vi "Arduino DAQ LabVIEW.vi"() -> ()   [LabVIEW 2020]
uses:
  <vilib>/MakerHub/LINX/Public/Peripherals/Analog/Analog Read N Chans.vi
  <vilib>/MakerHub/LINX/Public/Peripherals/Analog/Analog Read 1 Chan.vi
  <vilib>/MakerHub/LINX/Private/Local IO/LinxAnalogRead.vi
  <vilib>/MakerHub/LINX/Public/Utilities/Check Channel.vi
  <vilib>/MakerHub/LINX/Public/Utilities/Open Serial.vi
  <vilib>/MakerHub/LINX/Private/Utilties/Generate Error.vi
  <vilib>/MakerHub/LINX/LMH-LINX.lvlib
panel:
  out "Voltages":dbl[](array[numeric])
  in  "AI Channel(s)":u8[](array[numeric])
  out "Waveform Chart":dbl(graph)
  out "Voltage":dbl
  in  "Serial Port":refnum<visa-resource-name>="N/A"
  in  "Stop":bool
  in  "Analog Channel":u8
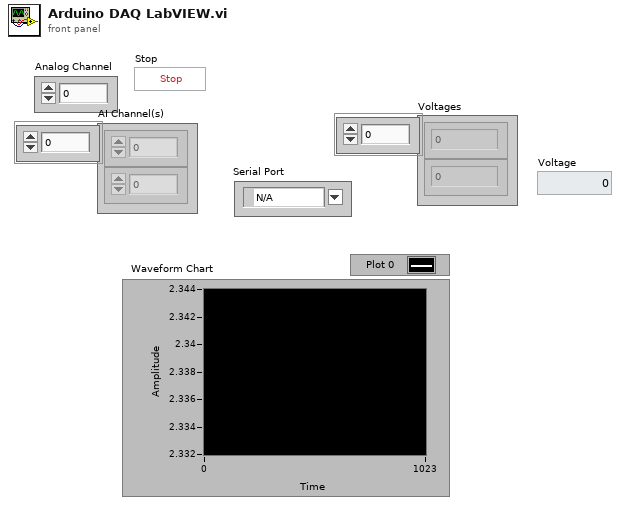
[diagram p1: front panel]
types:
  T1 = typedef "LMH-LINX.lvlib/LINX Ref.ctl" = cluster{"IO":T2, "Interface":T3, "LINX Device Config":T4}
  T2 = typedef "LMH-LINX.lvlib/Platform.ctl" = enum16{"Remote", "Local"}
  T3 = typedef "LMH-LINX.lvlib/Interface.ctl" = enum16{"Serial", "TCP"}
  T4 = typedef "LMH-LINX.lvlib/Device.lvlib/LINX Device Config.ctl" = cluster{"Interface":T3, "COM Port":refnum<visa-resource-name>, "TCP Configuration":T5, "Device Family":u8, "Device ID":u8, "Device Name":string, "TCP Ref":refnum<k5>, "Channels":T6}
  T5 = typedef "LMH-LINX.lvlib/Device.lvlib/TCP Config.ctl" = cluster{"IP Address":string, "Port":u16}
  T6 = typedef "LMH-LINX.lvlib/Channels.ctl" = cluster{"DI":u8[], "DO":u8[], "AI":u8[], "AO":u8[], "PWM":u8[], "QE":u8[], "UART":u8[], "I2C 2":u8[], "SPI":u8[], "CAN":u8[], "Servo":u8[], "AI Ref (V)":dbl, "AI Resolution (Bits)":u8, "AO Ref (V)":dbl, "AO Resolution (Bits)":u8}
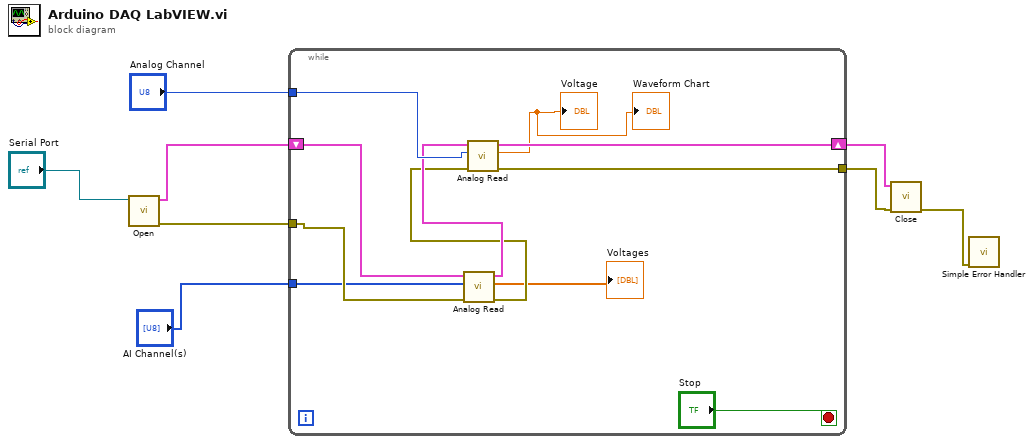
[diagram p0: block diagram]
diagram:
  n1 = call-poly <vilib>:"Open.vi"("Serial Port"="Serial Port") -> ("Error Out"=w7:errorcluster, "LINX Resource"=w8:T1)  [unwired: 8 in, 1 out]
  n2 = while {
    tunnel: w7 -> [w16]
    tunnel: "Analog Channel" -> [w18]
    tunnel: [w14] -> w2
    tunnel: "AI Channel(s)" -> [w10]
    shift-right: [w15] -> w3
    shift-left: w8 -> [w17]
    stop <- "Stop" stop-if-true
    n3 = call-poly <vilib>:"Analog Read.vi"("Error In"=w16, "AI Channel(s)"=w10, "LINX Resource"=w17) -> ("Error Out"=w11:errorcluster, "Voltages"=→"Voltages":dbl[], "LINX Resource"=w12:T1)  [unwired: 5 in, 1 out]
    n4 = call-poly <vilib>:"Analog Read.vi"("Error In"=w11, "Analog Channel"=w18, "LINX Resource"=w12) -> ("Error Out"=w14:errorcluster, "Voltage"=→"Voltage" →"Waveform Chart":dbl, "LINX Resource"=w15:T1)  [unwired: 5 in, 1 out]
  }
  n5 = call <vilib>:"Close.vi"("Error In"=w2, "LINX Resource"=w3) -> ("Error Out"=w5:errorcluster)  [unwired: 9 in]
  n6 = call <vilib>:"Simple Error Handler.vi"("error in (no error)"=w5) -> ()  [unwired: 4 in, 5 out]
